vi "DeviceWrite.vi"(4 "error in (no error)":errorcluster, 5 "Command":string, 6 "DeviceKey In":string, 7 "USBLib In":refnum<k24>) -> (0 "error out":errorcluster, 2 "DeviceKey Out":string, 3 "USBLib Out":refnum<k24>)   [LabVIEW 2009]
uses:
  C:/Samples/LabVIEW/UseDeviceKey/LabVIEW 2009/UseDeviceKey (with Device VIs)/UsbDllWrap.dll
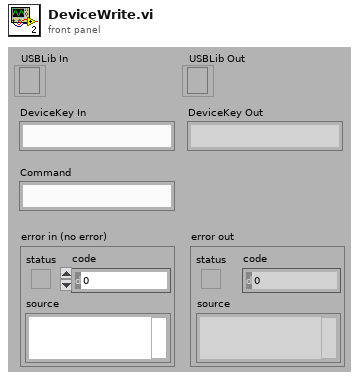
[diagram p1: front panel]
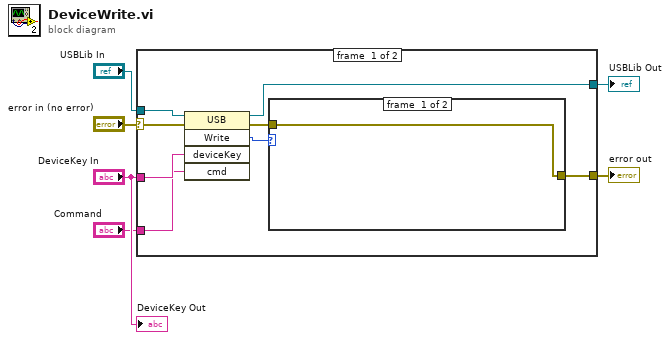
[diagram p0: block diagram]
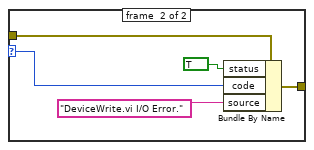
[diagram p2: hidden frame]
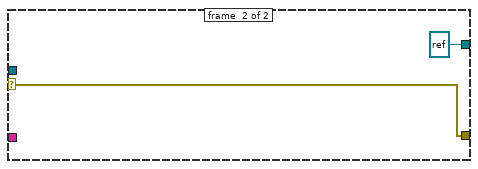
[diagram p3: hidden frame]
diagram:
  n1 = case shown="No Error" "error in (no error)" {
    selector: "error in (no error)" -> [w7 w22]
    tunnel: [w9 w22] -> w5
    tunnel: "DeviceKey In" -> [w14 _]
    tunnel: "Command" -> [w13 _]
    tunnel: "USBLib In" -> [w12 _]
    tunnel: [w11 refnum<k24> refnum ("USBLib In")] -> w1
    frame #0 {
      n2 = invoke class="USB" method="Write"(reference=w12, error in=w7, "deviceKey"=w14, "cmd"=w13) -> (reference out=w11:refnum<k24>, error out=w8:errorcluster, "Write"=w10:i32)  [unwired: 1 in, 2 out]
      n3 = case shown="1, Default" w10 {
        selector: w10 -> [_ w16]
        tunnel: w8 -> [w15 w18]
        tunnel: [w15 w17] -> w9
        frame #0 {
        }
        frame #1 {
          n4 = Bundle By Name(cluster=w18, "status"=TRUE, "code"=w16, "source"="DeviceWrite.vi I/O Error.") -> (w17:errorcluster)
        }
      }
    }
    frame #1 {
    }
  }
  "error out" <- w5
  "USBLib Out" <- w1
  "DeviceKey Out" <- "DeviceKey In"
